vi "Write to session log.vi"(1 "Session string":string="#Running Custom Tests") -> ()   [LabVIEW 2019]
uses:
  SiPM_Tests_Global_Var.vi
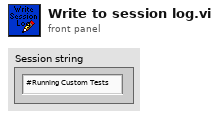
[diagram p1: front panel]
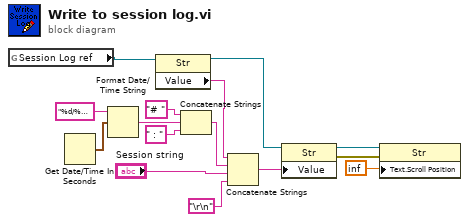
[diagram p0: block diagram]
diagram:
  n1 = global read "SiPM_Tests_Global_Var.vi" "Session Log ref"() -> (w4:refnum<vi>)
  n2 = Get Date/Time In Seconds() -> (seconds since 1Jan1904=w10:timestamp)
  n3 = Format Date/Time String(time format string (%c)="%d/%m/%y_%H:%M:%S", seconds (now)=w10) -> (date/time string=w12:string)  [unwired: 1 in]
  n4 = property on="Property Node" class="Str"(reference=w4) -> (reference out=w5:refnum<vi>, "Value"=w6:string)  [unwired: 1 in, 1 out]
  n5 = Concatenate Strings("# " ("string"), w12, " : " ("string")) -> (w15:string)
  n6 = Concatenate Strings(w6, w15, "Session string", "\r\n") -> (w7:string)
  n7 = property on="Property Node" class="Str"(reference=w5, "Value"=w7) -> (reference out=w2:refnum<vi>, error out=w1:errorcluster)  [unwired: 1 in]
  n8 = property on="Property Node" class="Str"(reference=w2, error in=w1, "Text.Scroll Position"=inf) -> ()  [unwired: 2 out]
